vi "Do Request.vi"(7 "Processing In":refnum<class "Processing.lvclass">, 11 "MCP Handler in":refnum<class "MCP Handler.lvclass">) -> (0 "error out":errorcluster, 5 "Processing":refnum<class "Processing.lvclass">)   [LabVIEW 2025, in "MCP Server.lvlib" / "MCP Handler.lvclass"]
doc: "A controller's main job is to respond to a request by generating a response. The response value must be specified by calling Set Response.vi on the Processing class that's passed through the VI otherwise an error will be generated.\n\nThere are several helpers available for common response types:\nGenerating HTML content programmatically - Create Basic Response.vi\nStreaming a file from disk - Create File Response.vi\nRedirecting the user to another URL - Create Redirect Response.vi\n\nFile responses are streamed in chunks and do not load the entire file into memory at once to send in the response which allows serving large files more efficiently."
uses:
  MCP Handler.lvclass
  <vilib>/IlluminatedG/IG HTTP Server/HTTP Server/Processing/Processing.lvclass
  <vilib>/IlluminatedG/IG HTTP Server/HTTP Server/Processing/Processing.lvclass/Processing.ctl
  MCP Handler.lvclass/MCP Handler.ctl
  <vilib>/IlluminatedG/IG HTTP Server/HTTP Server/Processing/Get Request.vi
  <vilib>/IlluminatedG/IG HTTP Utils/HTTP Utils/Request/Header Value.vi
  <vilib>/IlluminatedG/IG HTTP Utils/HTTP Utils/Request/Get Body.vi
  <vilib>/IlluminatedG/IG HTTP Utils/HTTP Utils/Response/Response.lvclass
  MCP Server.lvlib
panel:
  out "Exists":bool
  out "Value":string
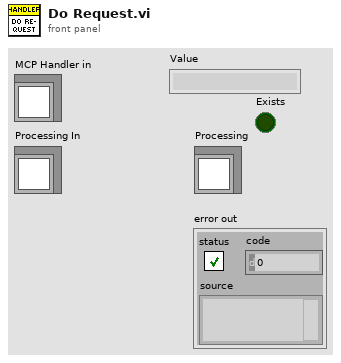
[diagram p1: front panel]
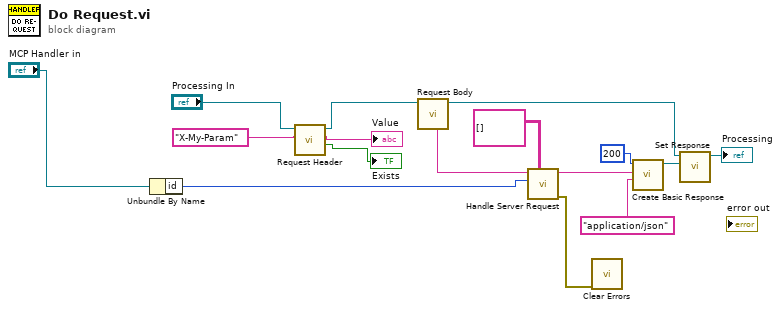
[diagram p0: block diagram]
diagram:
  n1 = Unbundle By Name("MCP Handler in") -> ("id"=w6:i32)
  n2 = call <vilib>:"Request Header.vi"("Header"="X-My-Param", "Processing in"="Processing In") -> ("Exists"=→"Exists":bool, "Value"=→"Value":string, "Processing out"=w3:refnum<class "Processing.lvclass">)  [unwired: 6 in, 1 out]
  n3 = call <vilib>:"Request Body.vi"("Processing in"=w3) -> ("Processing out"=w12:refnum<class "Processing.lvclass">, "Request Body"=w9:string)  [unwired: 9 in]
  n4 = call "Handle Server Request.vi"("parameters"=string[][] [], "id in"=w6, "request"=w9) -> ("error out"=w10:errorcluster, "response"=w8:string)  [unwired: 7 in]
  n5 = call <vilib>:"Clear Errors.vi"("error in (no error)"=w10) -> ()  [unwired: 5 in, 2 out]
  n6 = call <vilib>:"Create Basic Response.vi"("Content-Type (text/plain)"="application/json", "Payload"=w8, "Status Code"=u16 200) -> ("Response out"=w14:refnum<class "Response.lvclass">)  [unwired: 7 in, 1 out]
  n7 = call <vilib>:"Set Response.vi"("Response"=w14, "Processing in"=w12) -> ("Processing out"=→"Processing":refnum<class "Processing.lvclass">)  [unwired: 9 in]
